vi "read_attributes.vi"(8 "error in (no error)":errorcluster, 11 "MultiTaskLassoCV in":refnum<class "MultiTaskLassoCV.lvclass">) -> (0 "error out":errorcluster, 2 "attributes":T1, 3 "MultiTaskLassoCV out":refnum<class "MultiTaskLassoCV.lvclass">)   [LabVIEW 2020, in "MultiTaskLassoCV.lvclass"]
uses:
  MultiTaskLassoCV.lvclass
  Controls/multi_task_lasso_cv_attributes.ctl
  MultiTaskLassoCV.lvclass/MultiTaskLassoCV.ctl
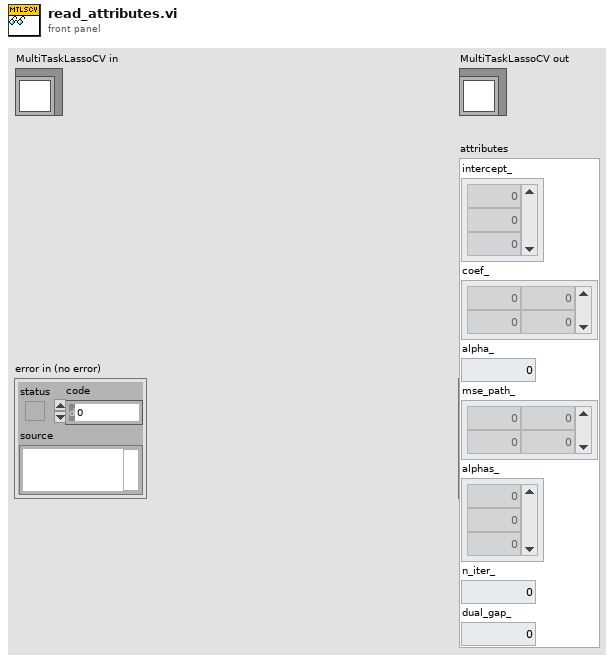
[diagram p1: front panel]
types:
  T1 = typedef "multi_task_lasso_cv_attributes.ctl" = cluster{"intercept_":dbl[], "coef_":dbl[][], "alpha_":dbl, "mse_path_":dbl[][], "alphas_":dbl[], "n_iter_":dbl, "dual_gap_":dbl}
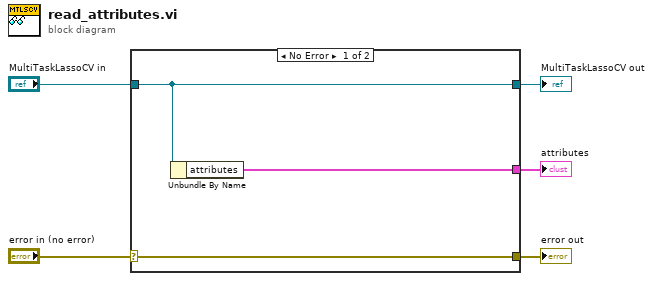
[diagram p0: block diagram]
diagram:
  n1 = case shown="No Error" "error in (no error)" {
    selector: "error in (no error)" -> [w8 w9]
    tunnel: [w8 w9] -> w4
    tunnel: [w7 w10] -> w2
    tunnel: "MultiTaskLassoCV in" -> [w7 w10]
    tunnel: [w6 _] -> w1
    frame No Error {
      n2 = Unbundle By Name(w7) -> ("attributes"=w6:T1)
    }
    frame Error {
    }
  }
  "error out" <- w4
  "MultiTaskLassoCV out" <- w2
  "attributes" <- w1
